vi "main01.vi"() -> ()   [LabVIEW 2018]
panel:
  out "ergebnis":dbl
  in  "b":dbl
  in  "a":dbl
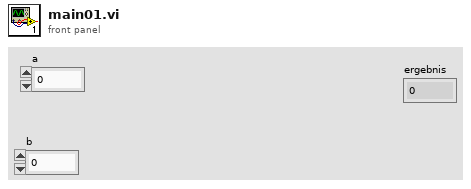
[diagram p1: front panel]
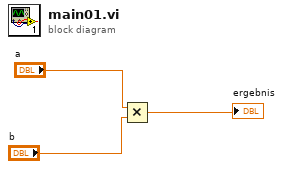
[diagram p0: block diagram]
diagram:
  n1 = Multiply(x="a", y="b") -> (x*y=→"ergebnis":dbl)
